vi "subject_Create.vi"(8 "error in (no error)":errorcluster, 10 "name":string, 11 "reference in":refnum<class "subject.lvclass">) -> (0 "error out":errorcluster, 3 "reference out":refnum<class "subject.lvclass">)   [LabVIEW 2015, in "subject.lvclass"]
doc: "Constructor."
uses:
  subject.lvclass
  <vilib>/addons/_AddQ/G#Object/utils/G#Object_CreateMethod.ctl
  <vilib>/addons/_AddQ/G#Object/G#Object.lvclass
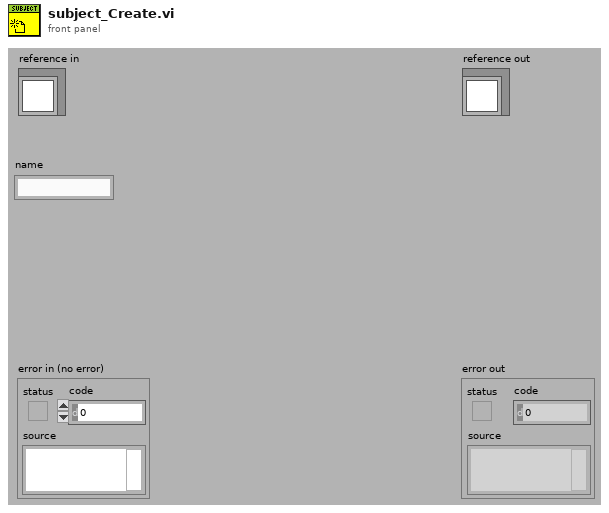
[diagram p1: front panel]
types:
  T1 = typedef "G#Object.lvclass/G#Object_CreateMethod.ctl" = enum16{"Create", "Create or look up existing", "Look up existing"}
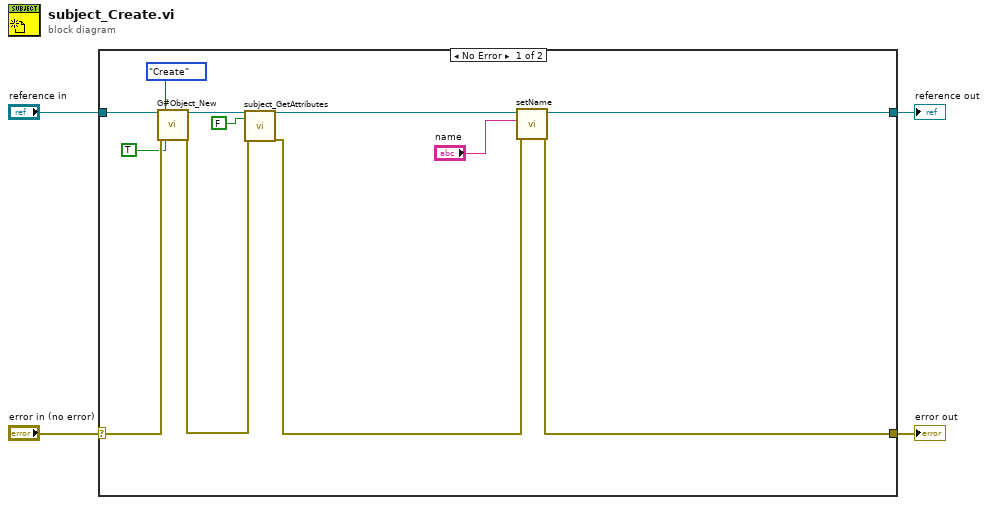
[diagram p0: block diagram]
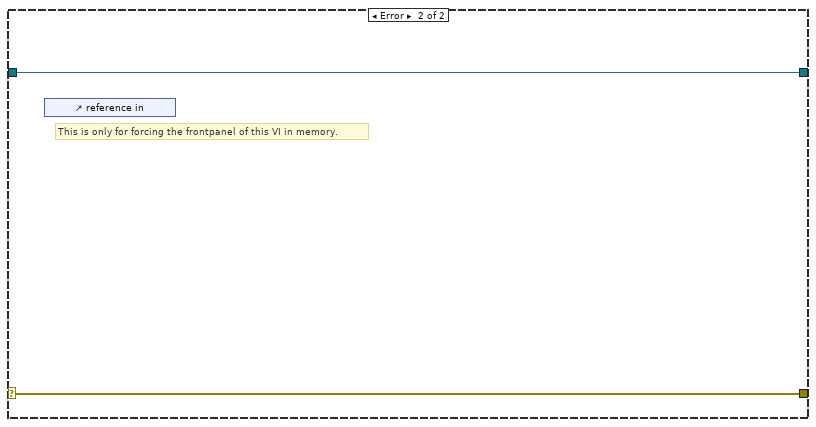
[diagram p2: hidden frame]
diagram:
  n1 = case shown="No Error" "error in (no error)" {
    selector: "error in (no error)" -> [w15 w18]
    tunnel: [w6 w18] -> w3
    tunnel: [w8 w17] -> w1
    tunnel: "reference in" -> [w16 w17]
    frame No Error {
      n2 = call <vilib>:"G#Object_New.vi"("reference in"=w16, "error in (no error)"=w15, "create method"=G#Object_CreateMethod."Create", "user counter (T)?"=TRUE ("User Counter")) -> ("reference out"=w13:refnum<class "subject.lvclass">, "error out"=w12:errorcluster)  [unwired: 13 in, 1 out]
      n3 = call "subject_GetAttributes.vi"("reference in"=w13, "return data? (T)"=FALSE ("return data"), "error in (no error)"=w12) -> ("reference out"=w9:refnum<class "subject.lvclass">, "error out"=w7:errorcluster)  [unwired: 13 in, 2 out]
      n4 = call "setName.vi"("error in (no error)"=w7, "name"="name", "reference in"=w9) -> ("error out"=w6:errorcluster, "reference out"=w8:refnum<class "subject.lvclass">)  [unwired: 7 in]
    }
    frame Error {
      # "This is only for forcing the frontpanel of this VI in memory."
      n5 = control-ref of="reference in"() -> ()  [unwired: 1 out]
    }
  }
  "error out" <- w3
  "reference out" <- w1
